vi "AI_OpenConfig.vi"(0 "SampleSettings":T3={"samples per channel"=100, "SampleRate"=1000.0, "TansMaxLength"=500000.0, "ReadTimeOut"=10.0, "时钟源"=""}, 1 "AI_ChannelSettings":T1 {"AI_SettingsArry"."标定系数"."Offset" format="%_4g"; "AI_SettingsArry"."标定系数"."Scale" format="%.4g"; "AI_SettingsArry"."shunt resistor location" items=["默认"=-1, "内部"=10200, "外部"=10167]; "AI_SettingsArry"."external shunt resistor value" format="%0.2f"; "AI_SettingsArry"."输入信号类型" items=["默认"=-1, "RSE"=10083, "NRSE"=10078, "差分"=10106, "伪差分"=12529]; "AI_SettingsArry"."单位" items=["安培"=10342, "伏特"=10348, "来自自定义换算"=10065]}, 5 "error in":errorcluster caption="错误输入") -> (14 "DAQ_AI_task_out":refnum<k21>, 19 "error out":errorcluster caption="错误输出")   [LabVIEW 2020, in "NI_DAQ.lvclass"]
uses:
  NI_DAQ.lvclass
  DAQ_Base_class/protected/SampleSettings.ctl
  DAQ_Base_class/protected/AI_ChannelSettings.ctl
  <vilib>/DAQmx/create/channels.llb/DAQmx Create Channel (AI-Voltage-Basic).vi
  <vilib>/DAQmx/create/channels.llb/DAQmx Create Channel (AI-Current-Basic).vi
  <vilib>/DAQmx/configure/timing.llb/DAQmx Timing (Sample Clock).vi
  DAQ_Base_class/DAQ_Base.lvclass
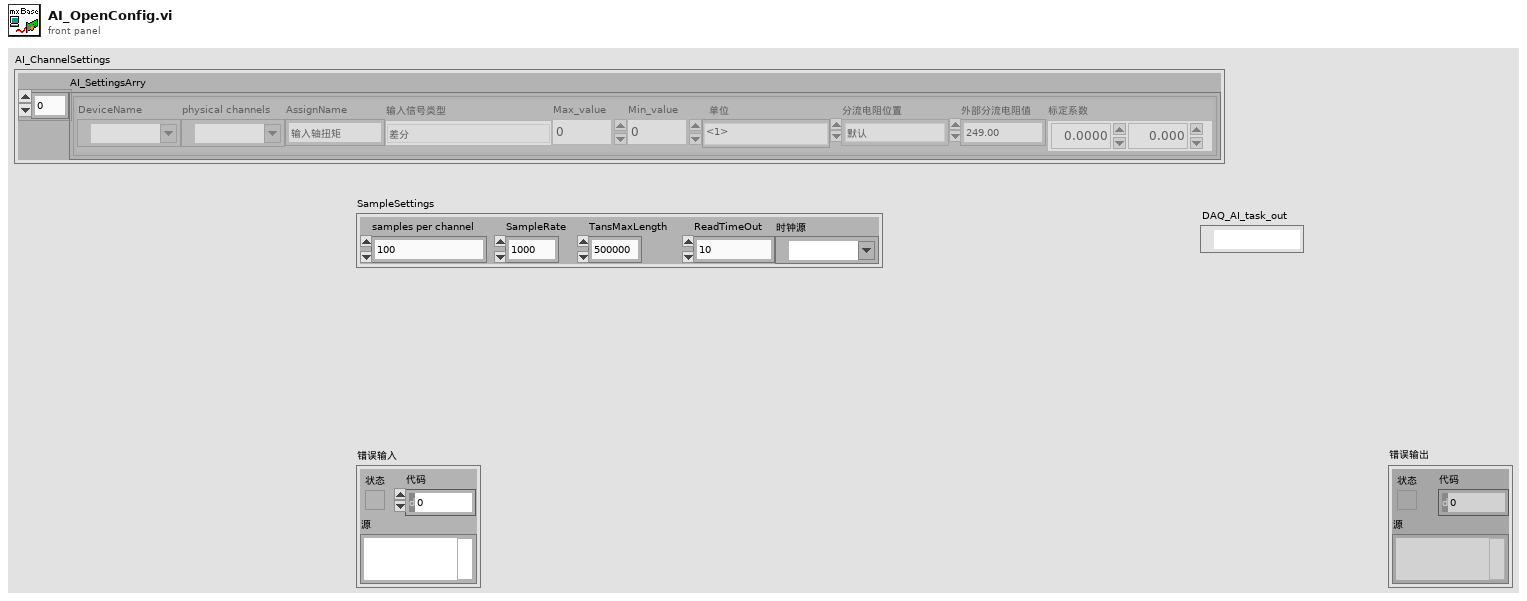
[diagram p1: front panel]
types:
  T1 = typedef "DAQ_Base.lvclass/AI_ChannelSettings.ctl" = cluster{"AI_SettingsArry":cluster{"DeviceName":tag, "physical channels":tag, "AssignName":string, "输入信号类型":T2, "Max_value":dbl, "Min_value":dbl, "单位":i32, "shunt resistor location":i32, "external shunt resistor value":dbl, "标定系数":cluster{"Scale":dbl, "Offset":dbl}}[]}
  T2 = typedef "AI信号类型.ctl" = i32
  T3 = typedef "DAQ_Base.lvclass/SampleSettings.ctl" = cluster{"samples per channel":i32, "SampleRate":dbl, "TansMaxLength":dbl, "ReadTimeOut":dbl, "时钟源":tag}
  T4 = cluster{"DeviceName":tag, "physical channels":tag, "AssignName":string, "输入信号类型":T2, "Max_value":dbl, "Min_value":dbl, "单位":i32, "shunt resistor location":i32, "external shunt resistor value":dbl, "标定系数":cluster{"Scale":dbl, "Offset":dbl}}[]
  T5 = cluster{"DeviceName":tag, "physical channels":tag, "AssignName":string, "输入信号类型":T2, "Max_value":dbl, "Min_value":dbl, "单位":i32, "shunt resistor location":i32, "external shunt resistor value":dbl, "标定系数":cluster{"Scale":dbl, "Offset":dbl}}
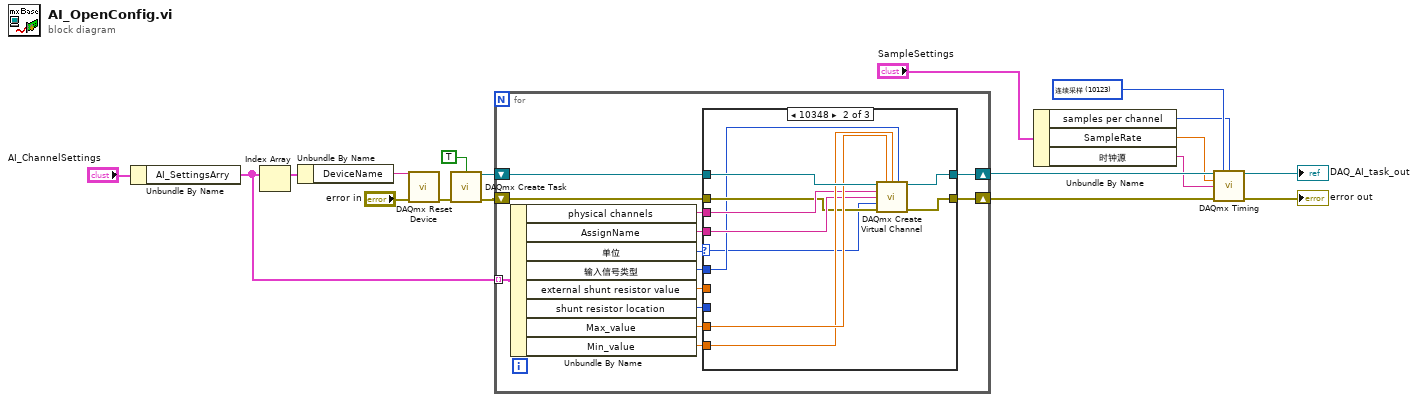
[diagram p0: block diagram]
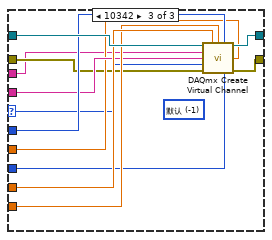
[diagram p3: hidden frame]
diagram:
  w16 = 10123 items=["有限采样"=10178, "连续采样"=10123, "硬件定时单点"=12522] ("sample mode")
  n1 = Unbundle By Name("AI_ChannelSettings") -> ("AI_SettingsArry"=w2:T4)
  n2 = Index Array(array=w2) -> (element=w10:T5)  [unwired: 1 in]
  n3 = Unbundle By Name(w10) -> ("DeviceName"=w9:tag)
  n4 = call <vilib>:"DAQmx Reset Device.vi"("device in"=w9, "error in"="error in") -> ("error out"=w12:errorcluster)  [unwired: 13 in]
  n5 = call <vilib>:"DAQmx Create Task.vi"("auto cleanup"=TRUE, "error in"=w12) -> ("task out"=w15:refnum<k21>, "error out"=w14:errorcluster)  [unwired: 3 in, 9 out]
  n6 = for {
    tunnel: w2 -> [w31] mode=indexing
    shift-right: [w28] -> w18
    shift-left: w15 -> [w29]
    shift-right: [w21] -> w17
    shift-left: w14 -> [w20]
    n7 = Unbundle By Name(w31) -> ("physical channels"=w30:tag, "AssignName"=w27:string, "单位"=w19:i32, "输入信号类型"=w26:T2, "external shunt resistor value"=w23:dbl, "shunt resistor location"=w22:i32, "Max_value"=w25:dbl, "Min_value"=w24:dbl)
    n8 = case shown="10348" w19 {
      selector: w19 -> [_ w34 w45]
      tunnel: w30 -> [_ w39 w46]
      tunnel: w29 -> [w33 w43 w55]
      tunnel: [w33 w42 w54] -> w28
      tunnel: w27 -> [_ w38 w50]
      tunnel: w26 -> [_ w35 w51]
      tunnel: w25 -> [_ w41 w53]
      tunnel: w24 -> [_ w40 w52]
      tunnel: w23 -> [_ _ w49]
      tunnel: w22 -> [_ _ w44]
      tunnel: [w32 w37 w47] -> w21
      tunnel: w20 -> [w32 w36 w48]
      frame Default {
      }
      frame 10348 {
        n9 = call-poly <vilib>:"DAQmx Create Virtual Channel.vi"("task in"=w43, "maximum value"=w41, "minimum value"=w40, "input terminal configuration"=w35, "physical channels"=w39, "name to assign"=w38, "units"=w34, "error in"=w36) -> ("task out"=w42:refnum<k21>, "error out"=w37:errorcluster)  [unwired: 6 in]
      }
      frame 10342 {
        (unwired) -1 items=["默认"=-1, "内部"=10200, "外部"=10167] ("shunt resistor location")
        n10 = call-poly <vilib>:"DAQmx Create Virtual Channel.vi"("task in"=w55, "maximum value"=w53, "minimum value"=w52, "input terminal configuration"=w51, "physical channels"=w46, "name to assign"=w50, "external shunt resistor value"=w49, "units"=w45, "error in"=w48, "shunt resistor location"=w44) -> ("task out"=w54:refnum<k21>, "error out"=w47:errorcluster)  [unwired: 4 in]
      }
    }
  }
  n11 = Unbundle By Name("SampleSettings") -> ("samples per channel"=w13:i32, "SampleRate"=w7:dbl, "时钟源"=w4:tag)
  n12 = call-poly <vilib>:"DAQmx Timing.vi"("task/channels in"=w18, "sample mode"=w16, "samples per channel"=w13, "rate"=w7, "source"=w4, "error in"=w17) -> ("task out"=→"DAQ_AI_task_out":refnum<k21>, "error out"=→"error out":errorcluster)  [unwired: 8 in]
